vi "Data - Receive.vi"() -> ()   [LabVIEW 2011]
uses:
  Data-Receive.ctl
panel:
  in  "Data Receive":T1
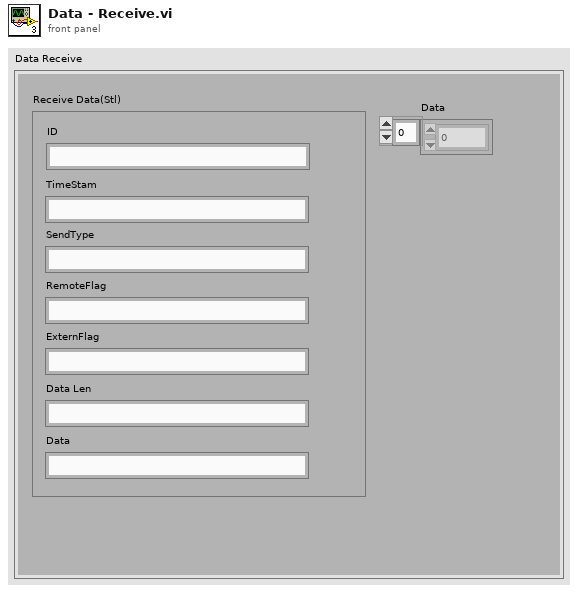
[diagram p1: front panel]
types:
  T1 = typedef "Data-Receive.ctl" = cluster{"Receive Data(Stl)":cluster{"TimeStam":string, "SendType":string, "RemoteFlag":string, "ExternFlag":string, "Data Len":string, "Data":string, "ID":string}, "Data":u8[]}
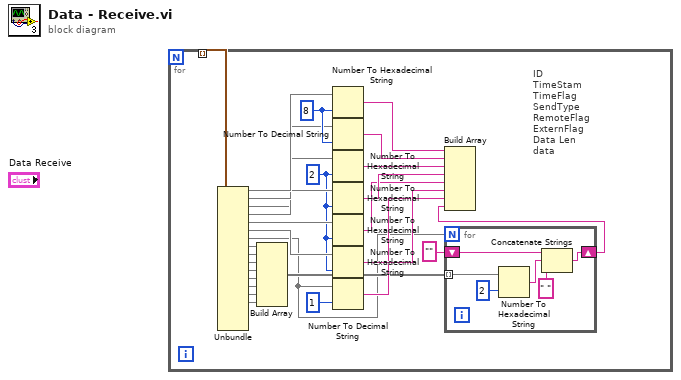
[diagram p0: block diagram]
diagram:
  n1 = for {
    tunnel: _ -> [w1] mode=indexing
    w6 = 2
    w27 = 8
    # "ID\nTimeStam\nTimeFlag\nSendType\nRemoteFlag\nExternFlag\nData Len\ndata"
    n2 = Unbundle(w1) -> ("ID"=w29, "TimeStamp"=w26, "TimeFlag"=w7, "SendType"=w24, "RemoteFlag"=w25, "ExternFlag"=w23, "DataLen"=w2, w16, w15, w14, w13, w12, w11, w9, w10)  [unwired: 3 out]
    n3 = Build Array(w16, w15, w14, w13, w12, w11, w9, w10) -> (w3:void[])
    n4 = Number To Hexadecimal String(1:w27, 2:w29) -> (0:w28:string)
    n5 = Number To Decimal String(number=w26, width (-)=w27) -> (decimal integer string=w22:string)
    n6 = Number To Hexadecimal String(1:w6, 2:w7) -> (0:w8:string)
    n7 = Number To Hexadecimal String(1:w6, 2:w24) -> (0:w21:string)
    n8 = Number To Hexadecimal String(1:w6, 2:w25) -> (0:w20:string)
    n9 = Number To Hexadecimal String(1:w6, 2:w23) -> (0:w19:string)
    n10 = Number To Decimal String(number=w2, width (-)=1) -> (decimal integer string=w17:string)
    n11 = for {
      N: w2 -> [_]
      shift-right: [w32] -> w5
      shift-left: "" -> [w30]
      tunnel: w3 -> [w31] mode=indexing
      n12 = Number To Hexadecimal String(1:i16 2 ("width (-)"), 2:w31) -> (0:w34:string)
      n13 = Concatenate Strings(w30, w34, " " ("string")) -> (w32:string)
    }
    n14 = Build Array(w28, w22, w8, w21, w20, w19, w17, w5) -> ()  [unwired: 1 out]
  }
